vi "Send Trigger.vi"(8 "error in (no error)":errorcluster, 11 "rfsa queue":refnum<queue>) -> (0 "error out":errorcluster)   [LabVIEW 2021]
uses:
  Messaging/RFSA Message.ctl
  RFSA Configuration.ctl
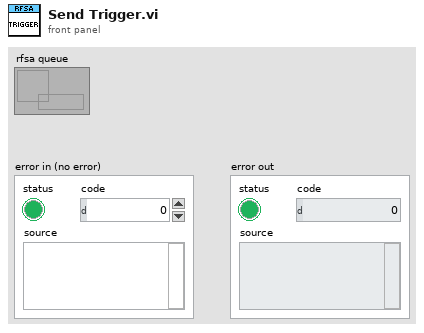
[diagram p1: front panel]
types:
  T1 = typedef "RFSA Message.ctl" = enum16{"Trigger Ready", "Run RF", "Stop RF", "Exit"}
  T2 = typedef "RFSA Configuration.ctl" = cluster{"rfsa ref":refnum<k15>, "cent freq":dbl, "iq rate":dbl, "power":dbl, "N/block":i64, "msg":T1}
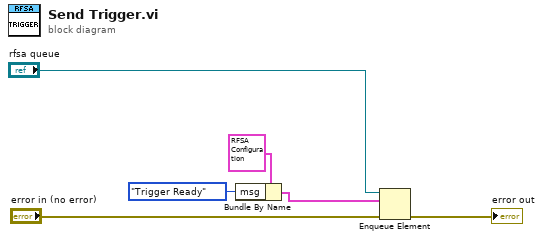
[diagram p0: block diagram]
diagram:
  n1 = Bundle By Name(cluster=T2 {"rfsa ref"="5646VST", "cent freq"=1000000000.0, "iq rate"=2000000.0, "power"=-10.0, "N/block"=1000, "msg"=enum."Trigger Ready"} ("element"), "msg"=RFSA_Message."Trigger Ready") -> (w1:T2)
  n2 = Enqueue Element(queue="rfsa queue", element=w1, error in (no error)="error in (no error)") -> (error out=→"error out":errorcluster)  [unwired: 1 in, 2 out]
